vi "writeSGLArray.vi"(8 "error in (no error)":errorcluster, 9 "Length":i32, 10 "Input":sgl[](array[numeric]), 11 "M1M3SAL in":refnum<class "M1M3SAL.lvclass">) -> (0 "error out":errorcluster, 3 "M1M3SAL out":refnum<class "M1M3SAL.lvclass">)   [LabVIEW 2016, in "M1M3SupportCommunicator.lvlib" / "M1M3SAL.lvclass"]
uses:
  M1M3SAL.lvclass
  M1M3SAL.lvclass/M1M3SAL.ctl
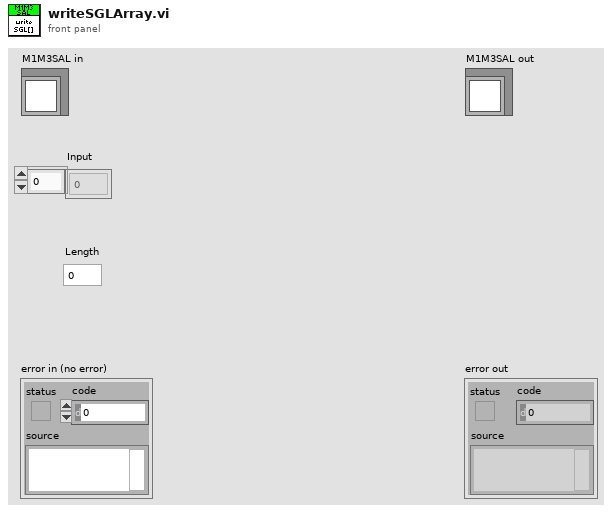
[diagram p1: front panel]
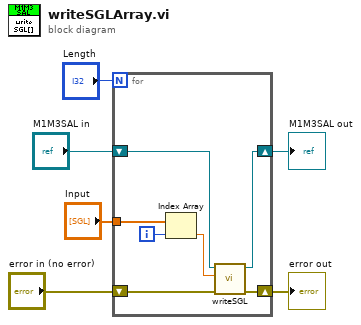
[diagram p0: block diagram]
diagram:
  n1 = for {
    N: "Length" -> [_]
    tunnel: "Input" -> [w13]
    shift-right: [w7] -> w3
    shift-left: "M1M3SAL in" -> [w11]
    shift-right: [w8] -> w1
    shift-left: "error in (no error)" -> [w9]
    i -> [w12]
    n2 = Index Array(array=w13, index=w12) -> (element=w10:sgl)
    n3 = call "writeSGL.vi"("error in (no error)"=w9, "Input"=w10, "M1M3SAL in"=w11) -> ("error out"=w8:errorcluster, "M1M3SAL out"=w7:refnum<class "M1M3SAL.lvclass">)  [unwired: 7 in]
  }
  "error out" <- w1
  "M1M3SAL out" <- w3
